vi "Get Values.vi"(8 "error in (no error)":errorcluster, 11 "EXFO in":refnum<class "EXFO.lvclass">) -> (0 "error out":errorcluster, 2 "Wavelength (nm)":dbl, 3 "EXFO out":refnum<class "EXFO.lvclass">, 5 "Attenuation":dbl, 7 "Power (uW)":dbl)   [LabVIEW 2018, in "LTB-1.lvlib" / "LTB-1.lvclass"]
uses:
  LTB-1.lvclass
  PPLs/EXFO/Parent/EXFO.lvlibp/EXFO.lvclass
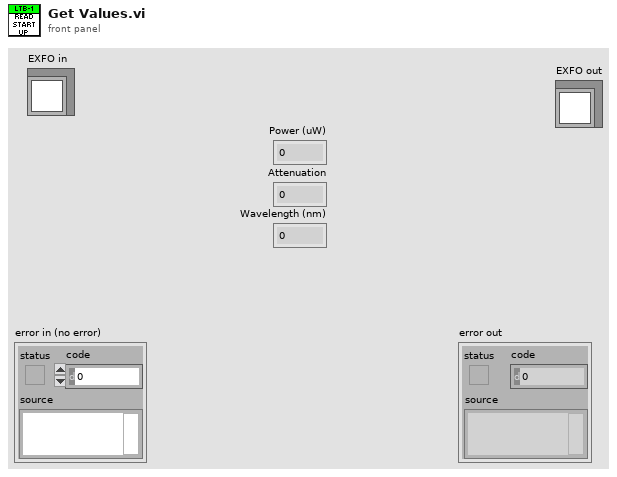
[diagram p1: front panel]
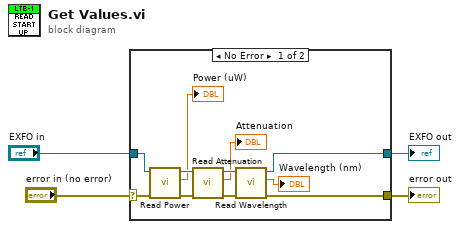
[diagram p0: block diagram]
diagram:
  n1 = case shown="No Error" "error in (no error)" {
    selector: "error in (no error)" -> [w9 w17]
    tunnel: [w8 w17] -> w3
    tunnel: [w12 w16] -> w2
    tunnel: "EXFO in" -> [w13 w16]
    frame No Error {
      n2 = call-dynamic "Read Power.vi"("error in (no error)"=w9, "EXFO in"=w13) -> ("error out"=w11:errorcluster, "Power (uW)"=→"Power (uW)":dbl, "EXFO out"=w15:refnum<class "EXFO.lvclass">)  [unwired: 6 in, 1 out]
      n3 = call-dynamic "Read Attenuation.vi"("error in (no error)"=w11, "EXFO in"=w15) -> ("error out"=w10:errorcluster, "Attenuation"=→"Attenuation":dbl, "EXFO out"=w14:refnum<class "EXFO.lvclass">)  [unwired: 7 in]
      n4 = call-dynamic "Read Wavelength.vi"("error in (no error)"=w10, "EXFO in"=w14) -> ("error out"=w8:errorcluster, "Wavelength (nm)"=→"Wavelength (nm)":dbl, "EXFO out"=w12:refnum<class "EXFO.lvclass">)  [unwired: 7 in]
    }
    frame Error {
    }
  }
  "error out" <- w3
  "EXFO out" <- w2
